vi "angle_iteration.vi"(1 "Phi":dbl, 2 "Goal Angle":dbl, 3 "Wind Vector":cluster{"Wind R":dbl, "Wind Theta":dbl}) -> (0 "Best Theta":dbl)   [LabVIEW 2011]
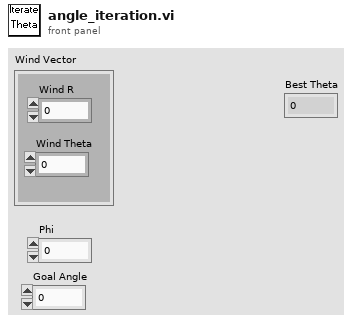
[diagram p1: front panel]
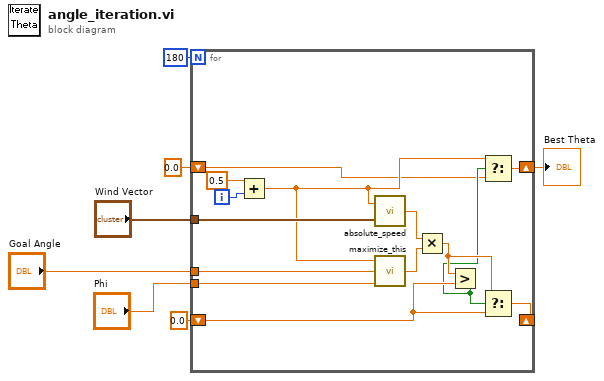
[diagram p0: block diagram]
diagram:
  n1 = for {
    N: 180 -> [_]
    tunnel: "Wind Vector" -> [w19]
    tunnel: "Phi" -> [w18]
    shift-right: [w14] -> _
    shift-left: 0.0 -> [w13]
    shift-right: [w10] -> w2
    shift-left: 0.0 -> [w9]
    tunnel: "Goal Angle" -> [w8]
    i -> [w21]
    n2 = Add(x=0.5, y=w21) -> (x+y=w11:dbl)
    n3 = call "absolute_speed.vi"("Wind Vector"=w19, "Boat Angle"=w11) -> ("Velocity"=w17:dbl)
    n4 = call "maximize_this.vi"("Phi"=w18, "Goal Angle"=w8, "Theta"=w11) -> ("Value"=w16:dbl)
    n5 = Multiply(x=w17, y=w16) -> (x*y=w15:dbl)
    n6 = Greater?(x=w15, y=w13) -> (0:w12:bool)
    n7 = Select(t=w11, s=w12, f=w9) -> (s? t:f=w10:dbl)
    n8 = Select(t=w15, s=w12, f=w13) -> (s? t:f=w14:dbl)
  }
  "Best Theta" <- w2
